vi "WSVCAP SHL Host TL I2C Write - Single Device.vi"(0 "Sub Address [U8]":u8=20 format="%.0x", 3 "FPGA":T1, 5 "Data Out [U8]":u8=20 format="%.0x", 11 "error in":errorcluster, 12 "DUT":T2, 13 "Device":T3, 14 "Log (T)":bool=TRUE) -> (15 "error out":errorcluster)   [LabVIEW 2012]
uses:
  Type Defs/WSVCAP SHL I2C Device Enum.ctl
  Type Defs/WSVCAP SHL DUT Number Enum.ctl
  Type Defs/WSVCAP SHL I2C FPGA Enum.ctl
panel:
  out "C3 Data Out [U8]":u8[](array[numeric]) format="%.0x"
  out "Socket Mask Set [U64]":u64[](array[numeric]) format="%012x"
  out "C2 Data Out [U8]":u8[](array[numeric]) format="%.0x"
  out "C1 Data Out [U8]":u8[](array[numeric]) format="%.0x"
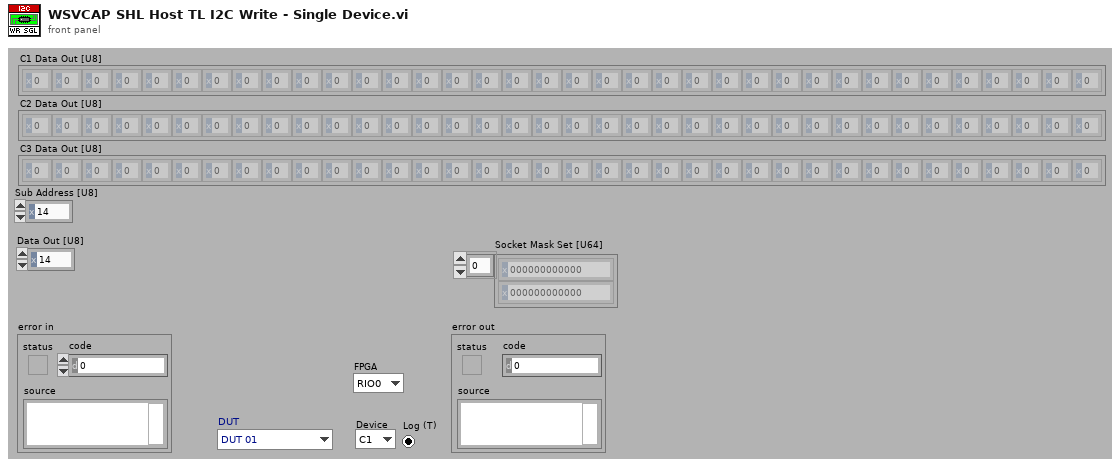
[diagram p1: front panel]
types:
  T1 = typedef "WSVCAP SHL I2C FPGA Enum.ctl" = enum16{"RIO0", "RIO1"}
  T2 = typedef "WSVCAP SHL DUT Number Enum.ctl" = enum16{"DUT 01", "DUT 02", "DUT 03", "DUT 04", "DUT 05", "DUT 06", "DUT 07", "DUT 08", "DUT 09", "DUT 10", "DUT 11", "DUT 12", "DUT 13", "DUT 14", "DUT 15", "DUT 16", "DUT 17", "DUT 18", "DUT 19", "DUT 20", "DUT 21", "DUT 22", "DUT 23", "DUT 24", "DUT 25", "DUT 26", "DUT 27", "DUT 28", "DUT 29", "DUT 30", "DUT 31", "DUT 32", "DUT 33", "DUT 34", "DUT 35", "DUT 36"}
  T3 = typedef "WSVCAP SHL I2C Device Enum.ctl" = enum16{"C1", "C2", "C3"}
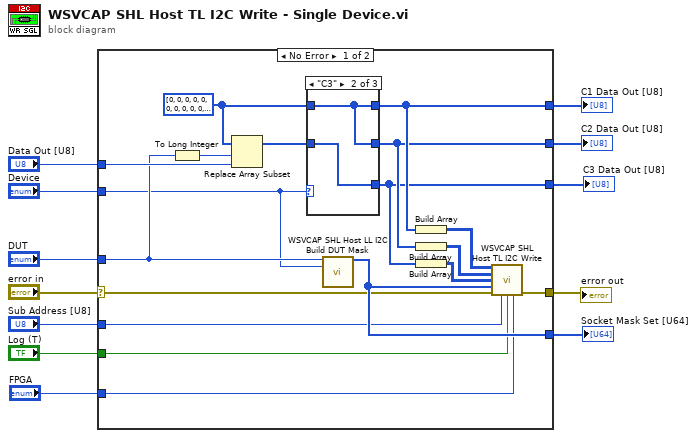
[diagram p0: block diagram]
diagram:
  n1 = case shown="No Error" "error in" {
    selector: "error in" -> [w19 w37]
    tunnel: [w30 w37] -> w12
    tunnel: "Sub Address [U8]" -> [w16 _]
    tunnel: "Data Out [U8]" -> [w29 _]
    tunnel: "Device" -> [w18 _]
    tunnel: [w23 _] -> w7
    tunnel: [w24 _] -> w6
    tunnel: "DUT" -> [w25 _]
    tunnel: [w20 _] -> w4
    tunnel: "Log (T)" -> [w17 _]
    tunnel: [w15 _] -> w2
    tunnel: "FPGA" -> [w13 _]
    frame No Error {
      w27 = u8[] [0, 0, 0, 0, 0, 0, 0, 0, 0, 0, 0, 0, 0, 0, 0, 0, 0, 0, 0, 0, 0, 0, 0, 0, 0, 0, 0, 0, 0, 0, 0, 0, 0, 0, 0, 0] ("SPI Data Out")
      n2 = To Long Integer(number=w25) -> (32bit integer=w28:i32)
      n3 = Replace Array Subset(array=w27, new element=w29, index=w28) -> (w26:u8[])
      n4 = case shown="\"C3\"" w18 {
        tunnel: [w31 w33 w36] -> w24
        tunnel: w27 -> [w31 w33 w35]
        tunnel: [w32 w33 w35] -> w23
        tunnel: w26 -> [w32 w34 w36]
        tunnel: [w31 w34 w35] -> w15
        frame "C2" {
        }
        frame "C3" {
        }
        frame "C1" {
        }
      }
      n5 = call "WSVCAP SHL Host LL I2C Build DUT Mask.vi"("DUT"=w25, "Device"=w18) -> ("Socket Mask Set [U64]"=w20:u64[])  [unwired: 12 in, 1 out]
      n6 = Build Array(w24) -> (w22:u8[][])
      n7 = Build Array(w23) -> (w21:u8[][])
      n8 = Build Array(w15) -> (w14:u8[][])
      n9 = call "WSVCAP SHL Host TL I2C Write.vi"("C1 Data Out"=w22, "C2 Data Out"=w21, "C3 Data Out"=w14, "Socket Mask Set [U64]"=w20, "error in"=w19, "Sub Address"=w16, "Log (T)"=w17, "FPGA"=w13) -> ("error out"=w30:errorcluster)  [unwired: 7 in]
    }
    frame Error {
    }
  }
  "error out" <- w12
  "C1 Data Out [U8]" <- w6
  "C2 Data Out [U8]" <- w7
  "Socket Mask Set [U64]" <- w4
  "C3 Data Out [U8]" <- w2
